vi "comDB.vi"(7 "error in (no error)":errorcluster caption="에러 입력(에러 없음)", 9 "Query":string, 10 "State":T1(ring)) -> (0 "error out":errorcluster caption="에러 출력", 1 "count":i64, 2 "result1DArray":string[](array[string]), 3 "resultList":string[][](table) caption="result2DArray")   [LabVIEW 2019]
uses:
  <vilib>/drjdpowell/SQLite Library/SQL Connection/Connection.lvclass
  <vilib>/drjdpowell/SQLite Library/SQL Connection/Open (string).vi
  <vilib>/drjdpowell/SQLite Library/SQLite.lvlib
  <vilib>/drjdpowell/SQLite Library/SQL Connection/Execute SQL (Single String).vi
  <vilib>/drjdpowell/SQLite Library/SQL Connection/Execute SQL.vi
  <vilib>/drjdpowell/SQLite Library/SQL Connection/Execute SQL (Single Integer).vi
  <vilib>/drjdpowell/SQLite Library/SQL Connection/Execute SQL (1D String).vi
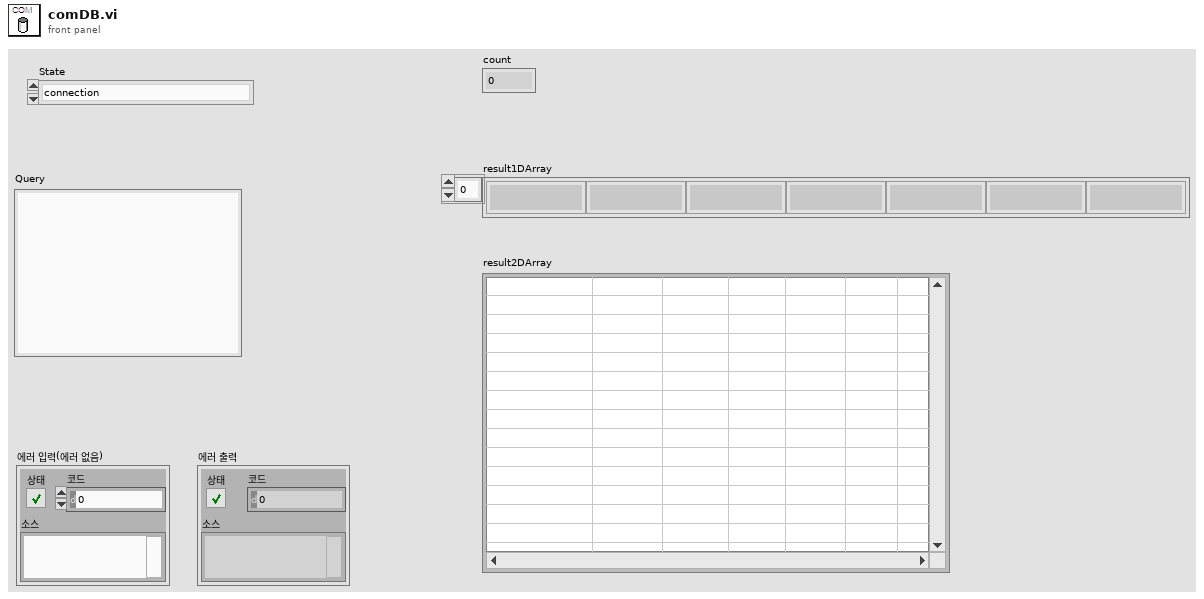
[diagram p1: front panel]
types:
  T1 = enum16{"connection", "create", "getReadList", "getRead", "getCount", "update", "delete", "close"}
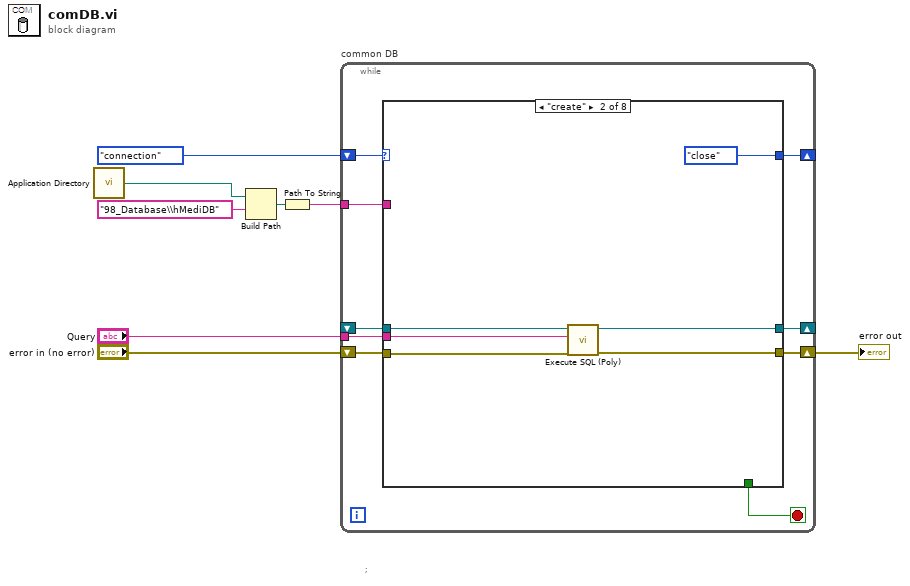
[diagram p0: block diagram]
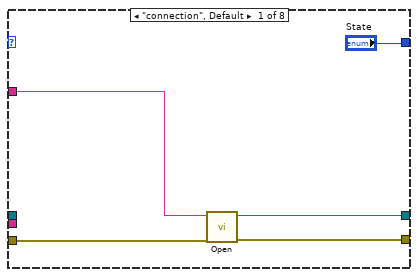
[diagram p2: hidden frame]
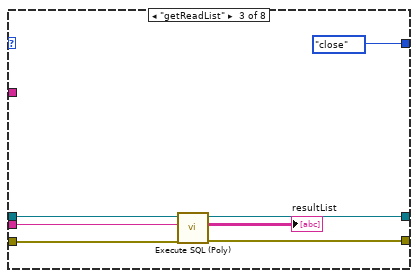
[diagram p3: hidden frame]
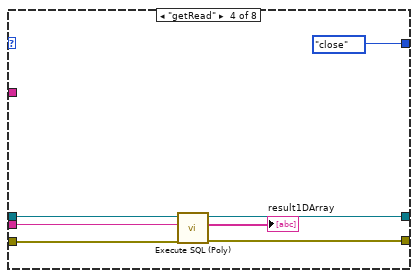
[diagram p4: hidden frame]
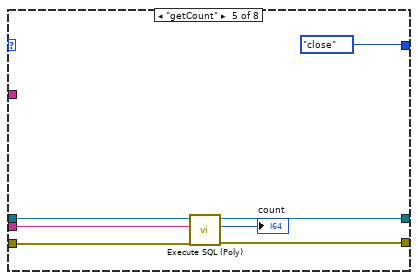
[diagram p5: hidden frame]
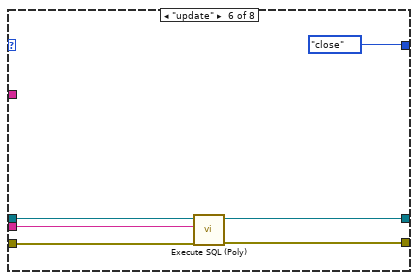
[diagram p6: hidden frame]
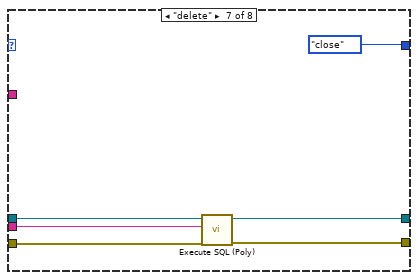
[diagram p7: hidden frame]
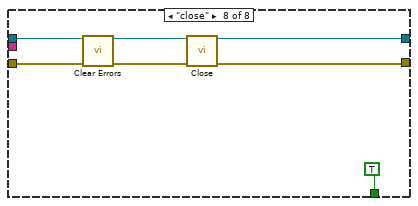
[diagram p8: hidden frame]
diagram:
  # ";"
  n1 = call <vilib>:"Application Directory.vi"() -> ("Application Directory"=w3:path)
  n2 = Build Path(base path=w3, name or relative path="98_Database\\hMediDB") -> (appended path=w2:path)
  n3 = Path To String(path=w2) -> (string=w1:string)
  n4 = while "common DB" {
    shift-right: [w16] -> _
    shift-left: _ -> [w15]
    tunnel: w1 -> [w13]
    shift-right: [w12] -> _
    shift-left: T1."connection" ("State") -> [w17]
    shift-right: [w14] -> w5
    shift-left: "error in (no error)" -> [w10]
    tunnel: "Query" -> [w9]
    stop <- w11 stop-if-true
    n5 = case shown="\"create\"" w17 {
      tunnel: [w22 w26 w33 w40 w47 w53 w59 w62] -> w16
      tunnel: w15 -> [_ w28 w35 w42 w49 w55 w61 w62]
      tunnel: [w21 w25 w32 w39 w46 w52 w58 w65] -> w14
      tunnel: w13 -> [w20 _ _ _ _ _ _ _]
      tunnel: w10 -> [w19 w27 w34 w41 w48 w54 w60 w66]
      tunnel: ["State" T1."close" ("State") T1."close" ("State") T1."close" ("State") T1."close" ("State") T1."close" ("State") T1."close" ("State") _] -> w12
      tunnel: [_ _ _ _ _ _ _ TRUE] -> w11
      tunnel: w9 -> [_ w24 w31 w38 w45 w51 w57 _]
      frame "connection", Default {
        n6 = call-poly <vilib>:"Open.vi"("error in (no error)"=w19, "db file"=w20) -> ("error out"=w21:errorcluster, "SQLite Connection"=w22:refnum<class "Connection.lvclass">)  [unwired: 8 in]
      }
      frame "create" {
        n7 = call-poly <vilib>:"Execute SQL (Poly).vi"("error in (no error)"=w27, "SQL"=w24, "SQLite Connection in"=w28) -> ("error out"=w25:errorcluster, "SQLite Connection"=w26:refnum<class "Connection.lvclass">)  [unwired: 6 in, 1 out]
      }
      frame "getReadList" {
        n8 = call-poly <vilib>:"Execute SQL (Poly).vi"("error in (no error)"=w34, "SQL"=w31, "SQLite Connection in"=w35) -> ("error out"=w32:errorcluster, "Result Set"=→"resultList":string[][], "SQLite Connection"=w33:refnum<class "Connection.lvclass">)  [unwired: 5 in, 1 out]
      }
      frame "getRead" {
        n9 = call-poly <vilib>:"Execute SQL (Poly).vi"("error in (no error)"=w41, "SQL"=w38, "SQLite Connection in"=w42) -> ("error out"=w39:errorcluster, "Result Set"=→"result1DArray":string[], "SQLite Connection"=w40:refnum<class "Connection.lvclass">)  [unwired: 5 in, 1 out]
      }
      frame "getCount" {
        n10 = call-poly <vilib>:"Execute SQL (Poly).vi"("error in (no error)"=w48, "SQL"=w45, "SQLite Connection in"=w49) -> ("error out"=w46:errorcluster, "Result"=→"count":i64, "SQLite Connection"=w47:refnum<class "Connection.lvclass">)  [unwired: 6 in]
      }
      frame "update" {
        n11 = call-poly <vilib>:"Execute SQL (Poly).vi"("error in (no error)"=w54, "SQL"=w51, "SQLite Connection in"=w55) -> ("error out"=w52:errorcluster, "SQLite Connection"=w53:refnum<class "Connection.lvclass">)  [unwired: 6 in, 1 out]
      }
      frame "delete" {
        n12 = call-poly <vilib>:"Execute SQL (Poly).vi"("error in (no error)"=w60, "SQL"=w57, "SQLite Connection in"=w61) -> ("error out"=w58:errorcluster, "SQLite Connection"=w59:refnum<class "Connection.lvclass">)  [unwired: 6 in, 1 out]
      }
      frame "close" {
        n13 = call <vilib>:"Clear Errors.vi"("error in (no error)"=w66) -> ("error out"=w63:errorcluster)  [unwired: 5 in, 1 out]
        n14 = call-dynamic "Close.vi"("error in (no error)"=w63, "SQLite Connection in"=w62) -> ("error out"=w65:errorcluster)  [unwired: 9 in]
      }
    }
  }
  "error out" <- w5
